vi "RT search for decimation channels.vi"(8 "error in (no error)":errorcluster, 10 "DataChan Type":T2, 11 "Device Reference":T1 format="%.0x") -> (0 "error out":errorcluster, 4 "FIFO Index Decimation Table":i32[](array[numeric])=[0, 2, 2, 0, 3], 6 "Block Address decimation table":u32[](array[numeric])=[0, 2, 2, 0, 3])   [LabVIEW 2017, in "RefMem DMA Custom Device.lvlib"]
uses:
  RefMem DMA Custom Device.lvlib
  Controls/Data Channel Type.ctl
  <vilib>/NI Veristand/Custom Device API/Custom Device Item Ref.ctl
  <vilib>/NI Veristand/Custom Device API/Get Item Property (U16).vi
  <vilib>/NI Veristand/Custom Device API/Get Item Property (U32).vi
  Controls/Global.vi
  <vilib>/NI Veristand/Custom Device Tools/Custom Device Utility Library/NI VeriStand - Search for All Items by GUID.vi
  <vilib>/NI VeriStand/Custom Device Tools/Custom Device Utility Library/Custom Device Utility Library.lvlib
  <vilib>/NI Veristand/Custom Device API/Custom Device API.lvlib
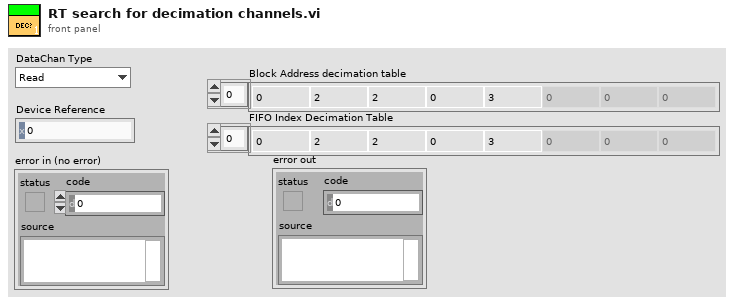
[diagram p1: front panel]
types:
  T1 = typedef "Custom Device API.lvlib/Custom Device Item Ref.ctl" = u64
  T2 = typedef "RefMem DMA Custom Device.lvlib/Data Channel Type.ctl" = enum16{"Read", "Write"}
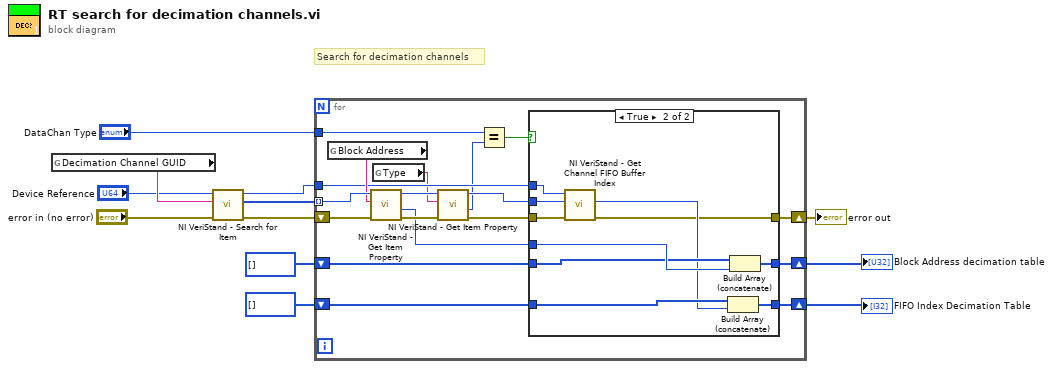
[diagram p0: block diagram]
diagram:
  # "Search for decimation channels"
  n1 = global read "Global.vi" "Decimation Channel GUID"() -> (w7:string)
  n2 = call-poly <vilib>:"NI VeriStand - Search for Item.vi"("error in"="error in (no error)", "Item GUID"=w7, "Section Ref in"="Device Reference") -> ("error out"=w11:errorcluster, "Item Refs"=w10:T1[], "Section Ref out"=w9:T1)  [unwired: 5 in, 1 out]
  n3 = for {
    tunnel: w9 -> [w27]
    tunnel: w10 -> [w30] mode=indexing
    shift-right: [w18] -> w1
    shift-left: i32[] [] ("Array") -> [w17]
    tunnel: "DataChan Type" -> [w20]
    shift-right: [w15] -> w2
    shift-left: u32[] [] ("Array") -> [w14]
    shift-right: [w13] -> w3
    shift-left: w11 -> [w29]
    n4 = global read "Global.vi" "Block Address"() -> (w28:string)
    n5 = call-poly <vilib>:"NI VeriStand - Get Item Property.vi"("error in (no error)"=w29, "Property Name"=w28, "Item Ref in"=w30) -> ("error out"=w25:errorcluster, "Value"=w16:u32, "Item Ref out"=w26:T1)  [unwired: 5 in, 1 out]
    n6 = global read "Global.vi" "Type"() -> (w22:string)
    n7 = call-poly <vilib>:"NI VeriStand - Get Item Property.vi"("error in (no error)"=w25, "Property Name"=w22, "Item Ref in"=w26) -> ("error out"=w24:errorcluster, "Value"=w21:u16, "Item Ref out"=w23:T1)  [unwired: 5 in, 1 out]
    n8 = Equal?(x=w20, y=w21) -> (x = y?=w19:bool)
    n9 = case shown="True" w19 {
      tunnel: w24 -> [w31 w43]
      tunnel: w27 -> [_ w42]
      tunnel: w23 -> [_ w41]
      tunnel: [w33 w36] -> w18
      tunnel: w17 -> [w33 w37]
      tunnel: w16 -> [_ w40]
      tunnel: [w32 w38] -> w15
      tunnel: w14 -> [w32 w39]
      tunnel: [w31 w34] -> w13
      frame False {
      }
      frame True {
        n10 = call <vilib>:"NI VeriStand - Get Channel FIFO Buffer Index.vi"("error in"=w43, "Channel Ref"=w41, "Device Ref in"=w42) -> ("error out"=w34:errorcluster, "Channel FIFO Buffer Index"=w35:i32)  [unwired: 4 in, 3 out]
        n11 = Build Array (concatenate)(w37, w35) -> (w36:i32[])
        n12 = Build Array (concatenate)(w39, w40) -> (w38:u32[])
      }
    }
  }
  "Block Address decimation table" <- w2
  "FIFO Index Decimation Table" <- w1
  "error out" <- w3
